vi "Simple Add.vi"(9 "Addend 3":dbl, 10 "Addend 2":dbl, 11 "Addend 1":dbl) -> (3 "Sum":dbl)   [LabVIEW 2020]
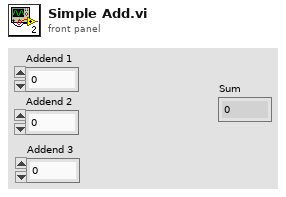
[diagram p1: front panel]
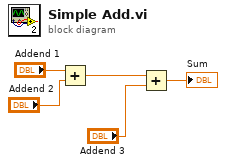
[diagram p0: block diagram]
diagram:
  n1 = Add(x="Addend 1", y="Addend 2") -> (x+y=w3:dbl)
  n2 = Add(x=w3, y="Addend 3") -> (x+y=→"Sum":dbl)
